vi "Build Frame Header.vi"(4 "Message Frame":T1) -> (7 "Header":string)   [LabVIEW 2020, in "HTTP Server.lvlib" / "WebSocket Client.lvclass"]
uses:
  WebSocket Client.lvclass
  WebSocket Client.lvclass/WebSocket Client.ctl
  OpCode.ctl
  Message Frame.ctl
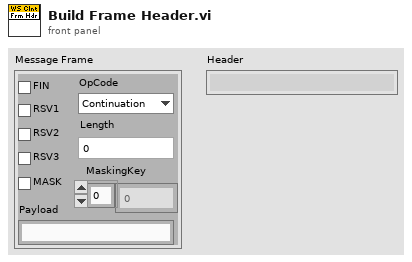
[diagram p1: front panel]
types:
  T1 = typedef "HTTP Server.lvlib/WebSocket Client.lvclass/Message Frame.ctl" = cluster{"FIN":bool, "RSV1":bool, "RSV2":bool, "RSV3":bool, "MASK":bool, "OpCode":T2, "Length":u64, "MaskingKey":u8[], "Payload":string}
  T2 = typedef "HTTP Server.lvlib/WebSocket Client.lvclass/OpCode.ctl" = enum8{"Continuation", "Text", "Binary", "Reserved3", "Reserved4", "Reserved5", "Reserved6", "Reserved7", "Close", "Ping", "Pong", "ReservedB", "ReservedC", "ReservedD", "ReservedE", "ReservedF"}
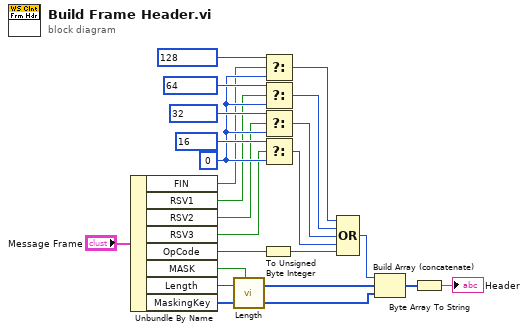
[diagram p0: block diagram]
diagram:
  w16 = u8 0
  n1 = Unbundle By Name("Message Frame") -> ("FIN"=w15:bool, "RSV1"=w14:bool, "RSV2"=w13:bool, "RSV3"=w12:bool, "OpCode"=w22:T2, "MASK"=w7:bool, "Length"=w6:u64, "MaskingKey"=w3:u8[])
  n2 = call "Length.vi"("Length"=w6, "Mask"=w7) -> ("Length Data"=w5:u8[])  [unwired: 5 in]
  n3 = To Unsigned Byte Integer(number=w22) -> (unsigned 8bit integer=w21:u8)
  n4 = Select(t=u8 128, s=w15, f=w16) -> (s? t:f=w8:u8)
  n5 = Select(t=u8 64, s=w14, f=w16) -> (s? t:f=w9:u8)
  n6 = Select(t=u8 32, s=w13, f=w16) -> (s? t:f=w10:u8)
  n7 = Select(t=u8 16, s=w12, f=w16) -> (s? t:f=w11:u8)
  n8 = Compound Arithmetic op=OR(w8, w9, w10, w11, w21) -> (w4:u8)
  n9 = Build Array (concatenate)(w4, w5, w3) -> (w2:u8[])
  n10 = Byte Array To String(unsigned byte array=w2) -> (string=→"Header":string)
